vi "Phasor Convert (tau, f) to (g, s) & (m, phi).vi"(8 "Error In":errorcluster, 9 "Phasor Frequency":dbl[unit], 11 "Phase Lifetime":dbl[unit]) -> (0 "Error Out":errorcluster, 1 "Phasor (m, phi)":T2, 3 "Phasor (g, s)":T1)   [LabVIEW 2021, in "Phasor.lvlib"]
uses:
  Phasor.lvlib
  Phasor (m, phi).ctl
  Phasor (g, s).ctl
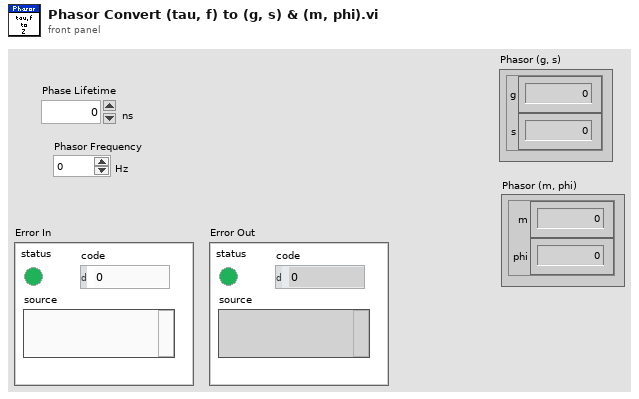
[diagram p1: front panel]
types:
  T1 = typedef "Phasor.lvlib/Phasor (g, s).ctl" = cluster{"g":dbl, "s":dbl}
  T2 = typedef "Phasor.lvlib/Phasor (m, phi).ctl" = cluster{"m":dbl, "phi":dbl}
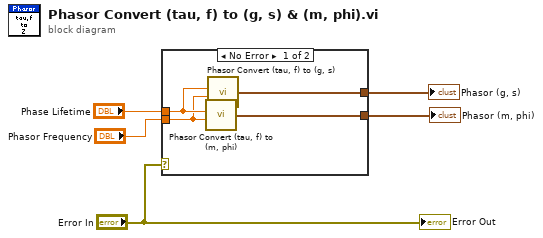
[diagram p0: block diagram]
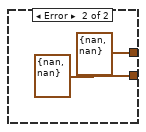
[diagram p2: hidden frame]
diagram:
  n1 = case shown="No Error" "Error In" {
    tunnel: "Phase Lifetime" -> [w8 _]
    tunnel: "Phasor Frequency" -> [w7 _]
    tunnel: [w9 T2 {"m"=nan, "phi"=nan} ("Phasor (m, phi)")] -> w3
    tunnel: [w6 T1 {"g"=nan, "s"=nan} ("Phasor (g, s)")] -> w2
    frame No Error {
      n2 = call "Phasor Convert (tau, f) to (m, phi).vi"("Lifetime"=w8, "Phasor Frequency"=w7) -> ("Phasor (m, phi)"=w9:T2)  [unwired: 5 in]
      n3 = call "Phasor Convert (tau, f) to (g, s).vi"("Lifetime"=w8, "Phasor Frequency"=w7) -> ("Phasor (g, s)"=w6:T1)  [unwired: 5 in]
    }
    frame Error {
    }
  }
  "Phasor (m, phi)" <- w3
  "Phasor (g, s)" <- w2
  "Error Out" <- "Error In"
